vi "Main Tclk.vi"() -> ()   [LabVIEW 2018] (continued)
      n7188 = local write "Faraday Cup array"(w9445) -> ()
      n7189 = local write "SEM Specimen I array"(w9445) -> ()
      n7190 = local write "Beam Dump 1 array"(w9445) -> ()
      n7191 = local write "Beam Dump 2 array"(w9445) -> ()
      n7192 = local write "Milling I array"(w9445) -> ()
      n7193 = local write "Focus index array"(w9445) -> ()
      n7194 = local write "Delta X array"(w9445) -> ()
      n7195 = local write "Delta Y array"(w9445) -> ()
      n7196 = local write "Specimen I array"(w9445) -> ()
      n7197 = case shown="2" w9444 {
        frame 0, Default {
        }
        frame 2 {
          n7198 = local read "Api"() -> (w9458:refnum<k7>)
          n7199 = call "SmartSEM Remote API set float.vi"("vValue"=sgl 0.0, "lpszParam"="DP_PANEL_DISABLE", "Api"=w9458) -> ("Api out"=w9454:refnum<k7>)  [unwired: 7 in, 1 out]
          n7200 = call "SmartSEM Remote API set float.vi"("vValue"=sgl 0.0, "lpszParam"="DP_JOYSTICK_DISABLE", "Api"=w9454) -> ()  [unwired: 7 in, 2 out]
        }
      }
      n7201 = local write "Temp high limit array"(w9445) -> ()
      n7202 = local write "Temp low limit array"(w9445) -> ()
      n7203 = local write "Specimen I high limit array"(w9445) -> ()
      n7204 = local write "Specimen I low limit array"(w9445) -> ()
      n7205 = local write "SEM Specimen I high limit array"(w9445) -> ()
      n7206 = local write "SEM Specimen I low limit array"(w9445) -> ()
      n7207 = local write "FI low limit array"(w9445) -> ()
      n7208 = local write "Faraday Cup high limit array"(w9445) -> ()
      n7209 = local write "Faraday Cup low limit array"(w9445) -> ()
      n7210 = local write "BD1 high limit array"(w9445) -> ()
      n7211 = local write "BD1 low limit array"(w9445) -> ()
      n7212 = local write "BD2 high limit array"(w9445) -> ()
      n7213 = local write "BD2 low limit array"(w9445) -> ()
      n7214 = local write "Milling I high limit array"(w9445) -> ()
      n7215 = local write "Milling I low limit array"(w9445) -> ()
    }
  }
